vi "PV ActiveLine - Protocol Serial Interface.vi"(7 "W/R":bool, 8 "Fehler (Eingang)":errorcluster, 9 "Protocol":i8(ring) items=["Auto", "PV Protocol", "Mnemonics"], 11 "Referenz in":refnum<visa-resource-name>) -> (0 "Cluster (Ausgang)":errorcluster, 1 "Read Status":u16(ring) items=["Read Failed", "Read Ok"], 2 "Protocol out":i8(ring) items=["Auto", "PV Protocol", "Mnemonics"], 3 "Referenz out":refnum<visa-resource-name>)   [LabVIEW 2013, in "PV ActiveLine.lvlib"]
doc: "PRO - Protocol Serial Interface\n\nTransmit: PRO [,a]\nReceive: a\n\nProtocol serial interface,\na =\n0 –> Automatic recognition (default)\n1 –> Pfeiffer Vacuum protocol\n2 –> Mnemonics protocol"
uses:
  <instrlib>/PV ActiveLine/PV ActiveLine.lvlib
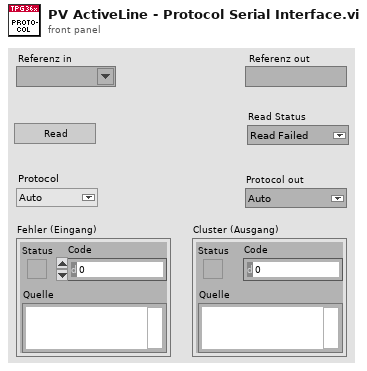
[diagram p1: front panel]
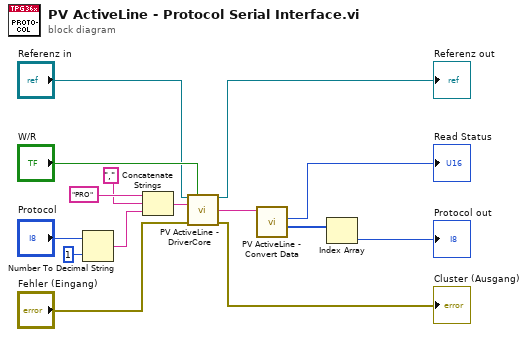
[diagram p0: block diagram]
diagram:
  n1 = Number To Decimal String(number="Protocol", width (-)=i16 1) -> (decimal integer string=w12:string)
  n2 = Concatenate Strings("PRO" ("Command"), "," ("Command"), w12) -> (w9:string)
  n3 = call <instrlib>:"PV ActiveLine - DriverCore.vi"("Referenz in"="Referenz in", "Write/Read"="W/R", "Command"=w9, "Fehler (Eingang)"="Fehler (Eingang)") -> ("Referenz out"=→"Referenz out":refnum<visa-resource-name>, "String Out"=w4:string, "Cluster (Ausgang)"=→"Cluster (Ausgang)":errorcluster)  [unwired: 9 in]
  n4 = call <instrlib>:"PV ActiveLine - Convert Data.vi"("String in"=w4) -> ("Integer Out"=w2:i32[], "Read Status"=→"Read Status":u16)  [unwired: 7 in, 2 out]
  n5 = Index Array(array=w2) -> (element=→"Protocol out":i32)  [unwired: 1 in]
